vi "SignalDisplay.vi"(3 "Channel Setting 1":T1 {"Meas Range" items=["-0.1 V~+0.1 V"=0.1, "-0.2 V~0.2 V"=0.2, "-0.5 V~+0.5 V"=0.5, "-1 V~+1 V"=1.0, "-2 V~+2 V"=2.0, "-5 V~+5 V"=5.0, "-10 V~+10 V"=10.0]; "Vertical\nPosition (Div)" min=-5.0 max=5.0 step=0.01 scale=-5.0..5.0 scale format="%.2f"; "Scale\n  Volts/Div" scale=0.01..20.0}, 4 "Double_Channel_Data_In":waveform(dbl)[](array[waveform]), 5 "Channel Setting 0":T1 {"Meas Range" items=["-0.1 V~+0.1 V"=0.1, "-0.2 V~0.2 V"=0.2, "-0.5 V~+0.5 V"=0.5, "-1 V~+1 V"=1.0, "-2 V~+2 V"=2.0, "-5 V~+5 V"=5.0, "-10 V~+10 V"=10.0]; "Vertical\nPosition (Div)" min=-5.0 max=5.0 step=0.01 scale=-5.0..5.0 scale format="%.2f"; "Scale\n  Volts/Div" scale=0.01..20.0}) -> (0 "Data_for_measure_out 1":waveform(dbl), 1 "波形图":waveform(dbl)[](graph), 2 "Data_for_measure_out 0":waveform(dbl))   [LabVIEW 2012]
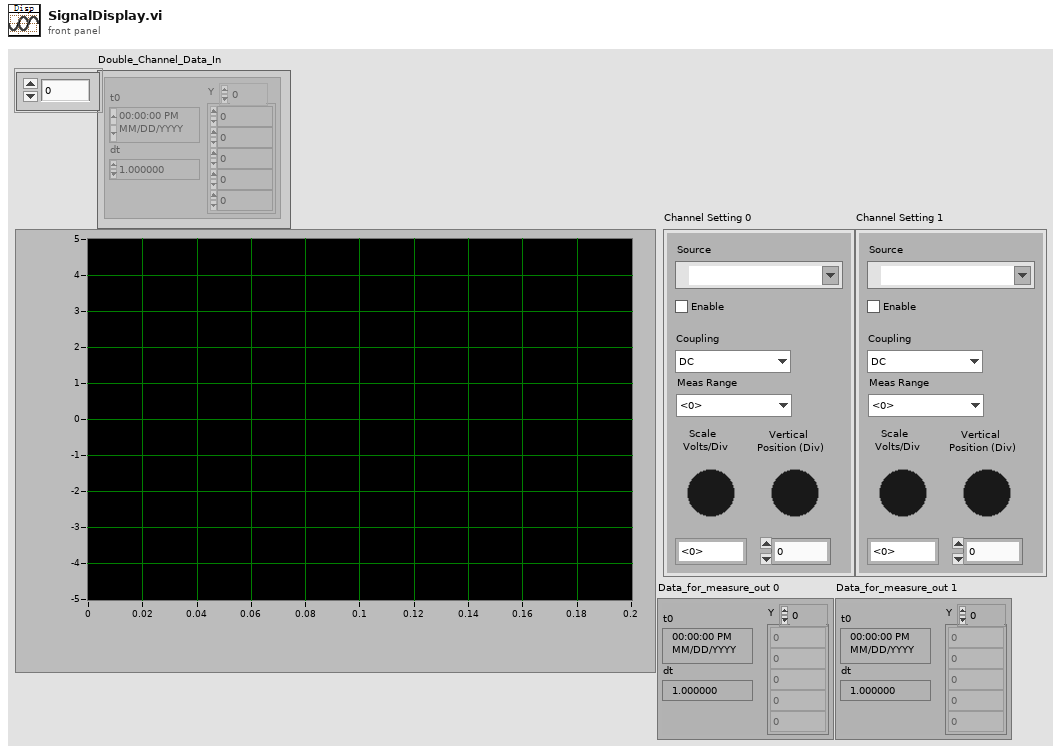
[diagram p1: front panel]
types:
  T1 = cluster{"physical channels":tag, "Enable":bool, "Coupling":enum16{"DC", "AC"}, "    Scale\n  Volts/Div  ":dbl, "    Vertical\nPosition (Div)":dbl, "Meas Range":dbl}
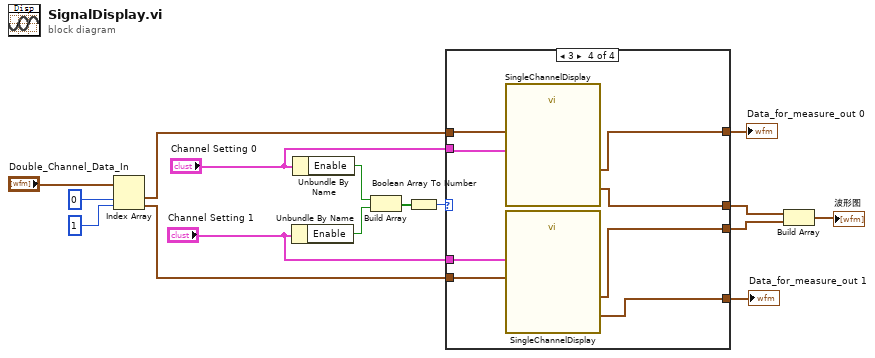
[diagram p0: block diagram]
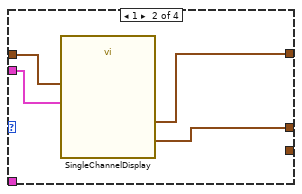
[diagram p3: hidden frame]
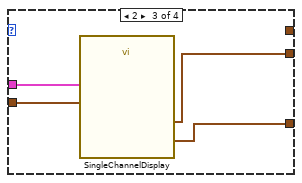
[diagram p4: hidden frame]
diagram:
  n1 = Index Array(array="Double_Channel_Data_In", index #1=0 ("索引 (行)"), index #2=1 ("索引")) -> (element #1=w7:waveform(dbl), element #2=w6:waveform(dbl))
  n2 = Unbundle By Name("Channel Setting 1") -> ("Enable"=w15:bool)
  n3 = Unbundle By Name("Channel Setting 0") -> ("Enable"=w16:bool)
  n4 = Build Array(w16, w15) -> (w14:bool[])
  n5 = Boolean Array To Number(Boolean array=w14) -> (number=w13:u32)
  n6 = case shown="3" w13 {
    tunnel: [_ _ w22 w26] -> w12
    tunnel: w7 -> [_ w20 _ w32]
    tunnel: w6 -> [_ _ w23 w27]
    tunnel: "Channel Setting 0" -> [_ w19 _ w31]
    tunnel: "Channel Setting 1" -> [_ _ w24 w28]
    tunnel: [_ w17 _ w29] -> w3
    tunnel: [_ w18 _ w30] -> w2
    tunnel: [_ _ w21 w25] -> w1
    frame 0, Default {
    }
    frame 1 {
      n7 = call "SingleChannelDisplay.vi"("Channel Setting"=w19, "Data In"=w20) -> ("Data_for_Display"=w17:waveform(dbl), "Data_for_measure_out"=w18:waveform(dbl))
    }
    frame 2 {
      n8 = call "SingleChannelDisplay.vi"("Channel Setting"=w24, "Data In"=w23) -> ("Data_for_Display"=w22:waveform(dbl), "Data_for_measure_out"=w21:waveform(dbl))
    }
    frame 3 {
      n9 = call "SingleChannelDisplay.vi"("Channel Setting"=w31, "Data In"=w32) -> ("Data_for_Display"=w29:waveform(dbl), "Data_for_measure_out"=w30:waveform(dbl))
      n10 = call "SingleChannelDisplay.vi"("Channel Setting"=w28, "Data In"=w27) -> ("Data_for_Display"=w26:waveform(dbl), "Data_for_measure_out"=w25:waveform(dbl))
    }
  }
  "Data_for_measure_out 0" <- w2
  "Data_for_measure_out 1" <- w1
  n11 = Build Array(w3, w12) -> (→"波形图":waveform(dbl)[])
